vi "JLINKARM EMU Select By USBSN.vi"(11 "SerialNo":u32) -> (3 "function return":i32)   [LabVIEW 2011, in "JLinkARM.lvlib"]
doc: "JLINKARMDLL_API int JLINKARM_EMU_SelectByUSBSN (U32 SerialNo);"
uses:
  Lib/JLinkARM.lvlib
  JLinkARM.dll
panel:
  out "error out":errorcluster
  in  "error in (no error)":errorcluster
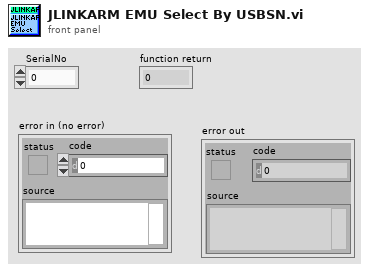
[diagram p1: front panel]
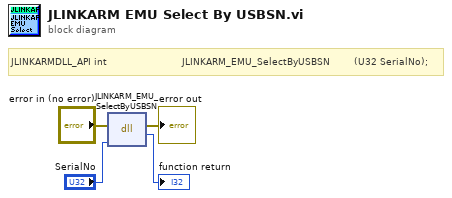
[diagram p0: block diagram]
diagram:
  # "JLINKARMDLL_API int                         JLINKARM_EMU_SelectByUSBSN        (U32 SerialNo);"
  n1 = dll-call lib="C:/Documents and Settings/Anybody/Desktop/JLink_SDK_V684a/JLinkARM.*" fn="JLINKARM_EMU_SelectByUSBSN"(error in="error in (no error)", "SerialNo"="SerialNo") -> (error out=→"error out":errorcluster, →"function return":i32)  [unwired: 3 in, 1 out]
